vi "_Obsolete_PathPlanner_Util_ReadJson.vi"(8 "error in (no error)":errorcluster, 11 "FileName":string="path1.path") -> (0 "error out":errorcluster, 3 "PathPlannerWayPoints":T1[](array[typedef]) {"HolonomicRotation"."SIN" format="%13.4f"; "HolonomicRotation"."COS" format="%13.4f"; "HolonomicRotation"."VALUE" format="%13.4f"; "NextControl"."Y" format="%14.3f"; "NextControl"."X" format="%14.3f"; "PrevControl"."Y" format="%14.3f"; "PrevControl"."X" format="%14.3f"; "AnchorPoint"."Y" format="%14.3f"; "AnchorPoint"."X" format="%14.3f"}, 4 "Full Filename":string)   [LabVIEW 2019, in "PathPlanner24.lvlib"]
doc: "Imports the Path Planner WayPoints from a JSON file.\n\nParameters:\n - FileName - File name string of the json file to import from\n - Error In - Error cluster (not used)\n\nReturns:\n - Trajectory - Trajectory data structure\n - Error out - Returned error cluster\n\nNote:\n -- Default path for roboRIO is /home/lvuser/natinst/LabVIEW Data\n -- Default path for Windows is: %USERPROFILE%\\Documents\\LabVIEW Data"
uses:
  PathPlanner24.lvlib
  TypeDef/PathPlannerWaypoint.ctl
  <vilib>/Rock Robotics/WPI/ThirdParty/JAS_Junk/TrajLib/TypeDef/TRANSLATION2D.ctl
  <vilib>/Rock Robotics/WPI/ThirdParty/JAS_Junk/TrajLib/TypeDef/ROTATION2D.ctl
  <vilib>/Rock Robotics/WPI/ThirdParty/JAS_Junk/TrajLib/Trajectory_Library.lvlib
panel:
  in  "Cluster":T4
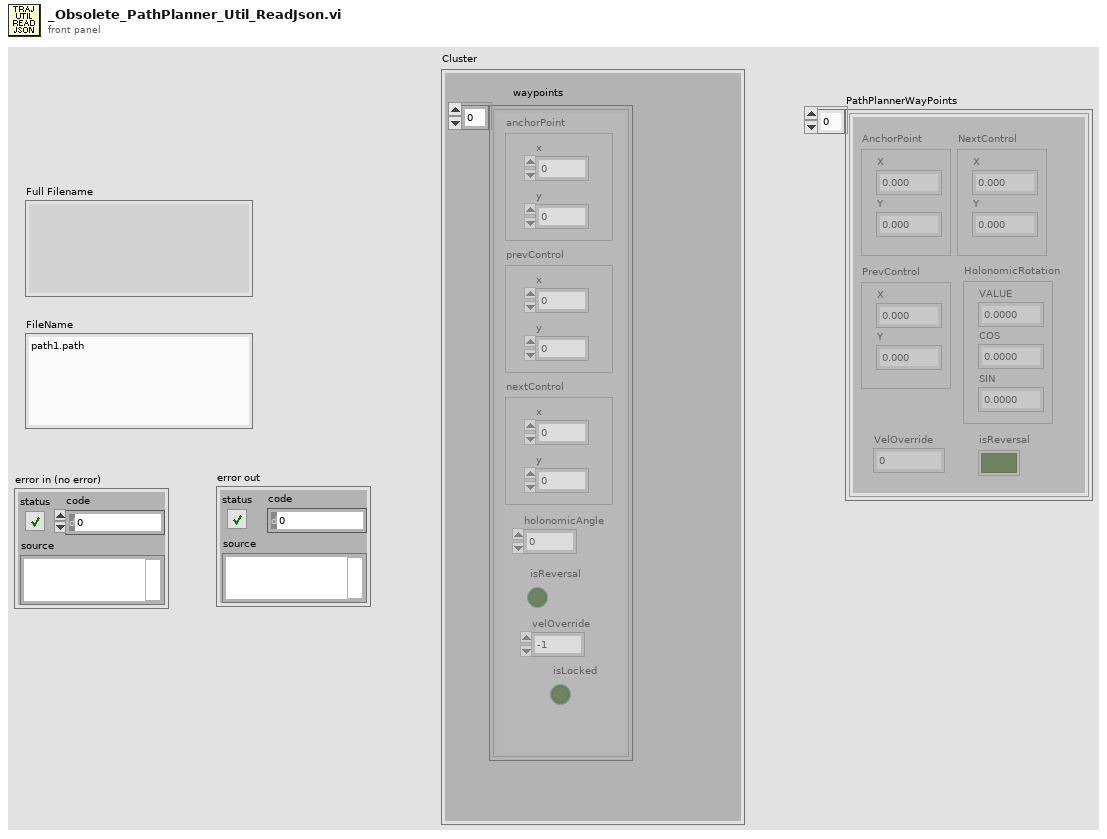
[diagram p1: front panel]
types:
  T1 = typedef "PathPlanner24.lvlib/PathPlannerWaypoint.ctl" = cluster{"AnchorPoint":T2, "PrevControl":T2, "NextControl":T2, "HolonomicRotation":T3, "VelOverride":dbl, "isReversal":bool}
  T2 = typedef "Trajectory_Library.lvlib/TRANSLATION2D.ctl" = cluster{"X":dbl, "Y":dbl}
  T3 = typedef "Trajectory_Library.lvlib/ROTATION2D.ctl" = cluster{"VALUE":dbl, "COS":dbl, "SIN":dbl}
  T4 = cluster{"waypoints":cluster{"anchorPoint":cluster{"x":dbl, "y":dbl}, "prevControl":cluster{"x":dbl, "y":dbl}, "nextControl":cluster{"x":dbl, "y":dbl}, "holonomicAngle":dbl, "isReversal":bool, "velOverride":dbl, "isLocked":bool}[]}
  T5 = enum16{"open", "replace", "create", "open or create", "replace or create", "replace or create with confirmation"}
  T6 = cluster{"anchorPoint":cluster{"x":dbl, "y":dbl}, "prevControl":cluster{"x":dbl, "y":dbl}, "nextControl":cluster{"x":dbl, "y":dbl}, "holonomicAngle":dbl, "isReversal":bool, "velOverride":dbl, "isLocked":bool}[]
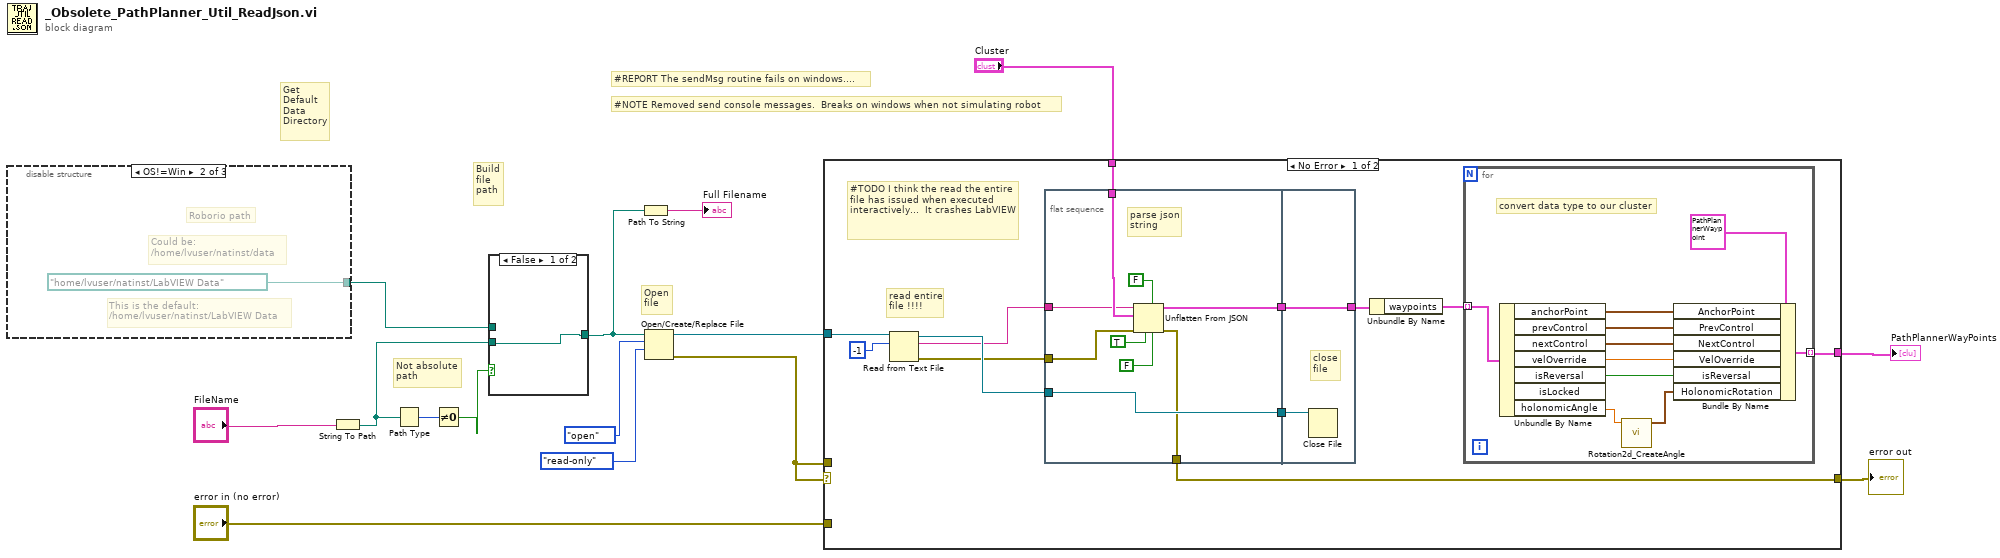
[diagram p0: block diagram]
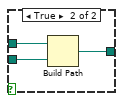
[diagram p2: hidden frame]
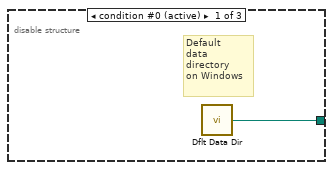
[diagram p3: hidden frame]
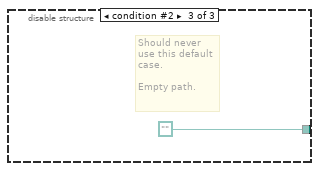
[diagram p4: hidden frame]
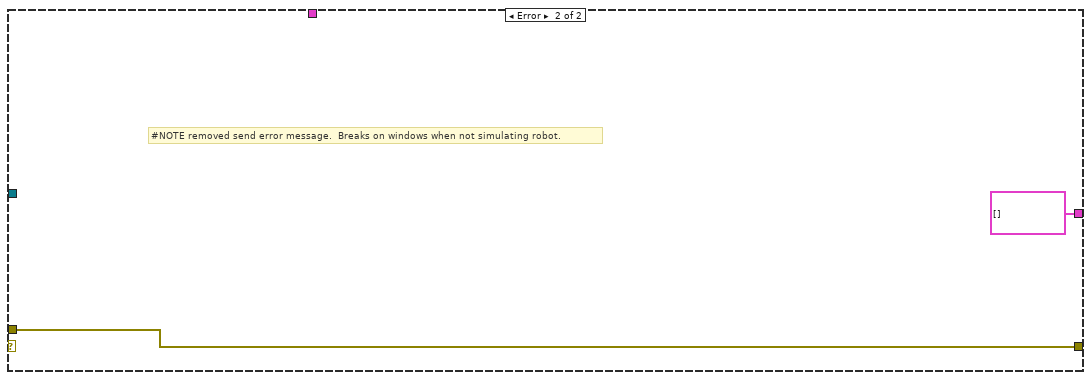
[diagram p5: hidden frame]
diagram:
  # "Not absolute\npath"
  # "#NOTE Removed send console messages.  Breaks on windows when not simulating robot"
  # "#REPORT The sendMsg routine fails on windows...."
  # "Get\nDefault\nData\nDirectory"
  # "Open\nfile"
  # "Build\nfile\npath"
  n1 = disable-structure shown="OS!=Win" {
    disable-tunnel: [w16 path "/home/lvuser/natinst/LabVIEW Data" path ""] -> w12
    frame condition #0 (active) {
      # "Default\ndata\ndirectory\non Windows"
      n2 = call <vilib>:"Dflt Data Dir.vi"() -> ("App:Default Data Directory"=w16:path)
    }
    frame condition #1 {
      # "This is the default:\n/home/lvuser/natinst/LabVIEW Data"
      # "Could be:\n/home/lvuser/natinst/data"
      # "Roborio path"
    }
    frame condition #2 {
      # "Should never\nuse this default\ncase.\n\nEmpty path."
    }
  }
  n3 = String To Path(string="FileName") -> (path=w10:path)
  n4 = Path Type(1:w10) -> (0:w9:i16)
  n5 = Not Equal To 0?(x=w9) -> (x != 0?=w8:bool)
  n6 = case shown="False" w8 {
    tunnel: [w19 w22] -> w4
    tunnel: w12 -> [_ w21]
    tunnel: w10 -> [w19 w20]
    frame False {
    }
    frame True {
      n7 = Build Path(base path=w21, name or relative path=w20) -> (appended path=w22:path)
    }
  }
  n8 = Path To String(path=w4) -> (string=→"Full Filename":string)
  n9 = Open/Create/Replace File(file path (use dialog)=w4, operation (0:open)=T5."open", access (0:read/write)=enum16{"read/write", "read-only", "write-only"}."read-only") -> (refnum out=w5:refnum<file>, error out=w13:errorcluster)  [unwired: 3 in, 1 out]
  n10 = case shown="No Error" w13 {
    tunnel: w5 -> [w33 _]
    tunnel: [w30 T1[] []] -> w1
    tunnel: w13 -> [_ w57]
    tunnel: [w29 w57] -> w7
    tunnel: "error in (no error)" -> [_ _]
    tunnel: "Cluster" -> [w27 _]
    frame No Error {
      # "#TODO I think the read the entire\nfile has issued when executed\ninteractively...  It crashes LabVIEW"
      # "read entire\nfile !!!!"
      n11 = Read from Text File(file (use dialog)=w33, count=-1) -> (refnum out=w32:refnum<file>, text=w26:string, error out=w28:errorcluster)  [unwired: 2 in, 1 out]
      n12 = flat-sequence {
        tunnel: w32 -> [w53]
        tunnel: [w53] -> w31
        tunnel: [w52] -> w29
        tunnel: w28 -> [w51]
        tunnel: w27 -> [w47]
        tunnel: w26 -> [w46]
        tunnel: [w45] -> w25
        tunnel: w31 -> [w55]
        tunnel: [w54] -> w24
        tunnel: w25 -> [w54]
        frame #0 {
          # "parse json\nstring"
          n13 = Unflatten From JSON(enable LabVIEW extensions? (T)=FALSE, JSON string=w46, type and defaults=w47, default null elements? (F)=TRUE, strict validation? (F)=FALSE, error in (no error)=w51) -> (value=w45:T4, error out=w52:errorcluster)  [unwired: 1 in]
        }
        frame #1 {
          # "close\nfile"
          n14 = Close File(refnum=w55) -> ()  [unwired: 1 in, 2 out]
        }
      }
      n15 = Unbundle By Name(w24) -> ("waypoints"=w23:T6)
      n16 = for {
        tunnel: [w43] -> w30 mode=indexing
        tunnel: w23 -> [w42] mode=indexing
        # "convert data type to our cluster"
        n17 = Unbundle By Name(w42) -> ("anchorPoint"=w41:cluster{"x":dbl, "y":dbl}, "prevControl"=w40:cluster{"x":dbl, "y":dbl}, "nextControl"=w39:cluster{"x":dbl, "y":dbl}, "velOverride"=w38:dbl, "isReversal"=w37:bool, "holonomicAngle"=w36:dbl)  [unwired: 1 out]
        n18 = call <vilib>:"Rotation2d_CreateAngle.vi"("Angle"=w36) -> ("ROTATION"=w35:T3)  [unwired: 10 in]
        n19 = Bundle By Name(cluster=T1 {"AnchorPoint"={"X"=0.0, "Y"=0.0}, "PrevControl"={"X"=0.0, "Y"=0.0}, "NextControl"={"X"=0.0, "Y"=0.0}, "HolonomicRotation"={"VALUE"=0.0, "COS"=1.0, "SIN"=0.0}, "VelOverride"=0.0, "isReversal"=FALSE} ("PathPlannerWaypoint"), "AnchorPoint"=w41, "PrevControl"=w40, "NextControl"=w39, "VelOverride"=w38, "isReversal"=w37, "HolonomicRotation"=w35) -> (w43:T1)
      }
    }
    frame Error {
      # "#NOTE removed send error message.  Breaks on windows when not simulating robot."
    }
  }
  "error out" <- w7
  "PathPlannerWayPoints" <- w1
